vi "SVE-Manager.vi"(9 "Data":variant, 10 "DataTag":string) -> (1 "error out":errorcluster)   [LabVIEW 2017]
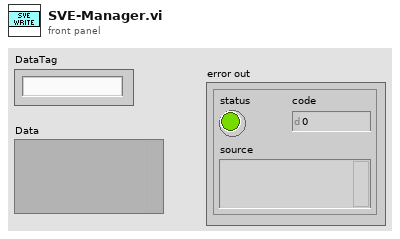
[diagram p1: front panel]
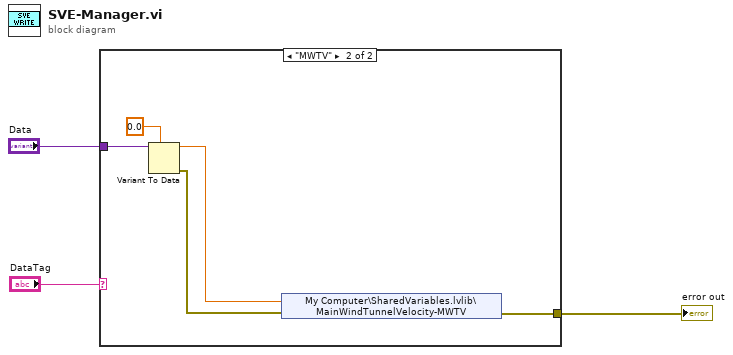
[diagram p0: block diagram]
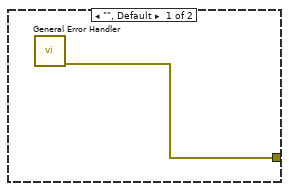
[diagram p2: hidden frame]
diagram:
  n1 = case shown="\"MWTV\"" "DataTag" {
    tunnel: [w4 w9] -> w2
    tunnel: "Data" -> [_ w7]
    frame "", Default {
      n2 = call <vilib>:"General Error Handler.vi"() -> ("error out"=w4:errorcluster)  [unwired: 11 in, 4 out]
    }
    frame "MWTV" {
      n3 = Variant To Data(type=0.0 ("MainWindTunnelVelocity-MWTV"), Variant=w7) -> (data=w6:dbl, error out=w5:errorcluster)  [unwired: 1 in]
      n4 = shared-variable "My Computer\\SharedVariables.lvlib\\MainWindTunnelVelocity-MWTV"(w6, error in=w5) -> (error out=w9:errorcluster)
    }
  }
  "error out" <- w2
